vi "insertTubel.vi"(8 "error in (no error)":errorcluster, 9 "Data Cluster":T1, 10 "Name of Table":string, 11 "DataCollector in":refnum<class "DataCollector.lvclass">) -> (0 "error out":errorcluster, 3 "DataCollector out":refnum<class "DataCollector.lvclass">)   [LabVIEW 2017, in "DataCollector.lvclass"]
uses:
  DataCollector.lvclass
  DataCollector.lvclass/DataCollector.ctl
  <vilib>/drjdpowell/SQLite Library/SQL Statement/SQL Statement.lvclass/SQL Statement.ctl
  <vilib>/drjdpowell/SQLite Library/SQL Statement/Bind Integer.vi
  <vilib>/drjdpowell/SQLite Library/SQL Statement/Bind Null.vi
  <vilib>/drjdpowell/SQLite Library/SQL Statement/Step.vi
  <vilib>/drjdpowell/SQLite Library/SQL Statement/Error Message.vi
  <vilib>/drjdpowell/SQLite Library/SQL Connection/Connection.lvclass
  <vilib>/drjdpowell/SQLite Library/SQL Statement/SQL Statement.lvclass
  <vilib>/drjdpowell/SQLite Library/Transaction Helpers/Transaction.lvlib
panel:
  out "concatenated string":string
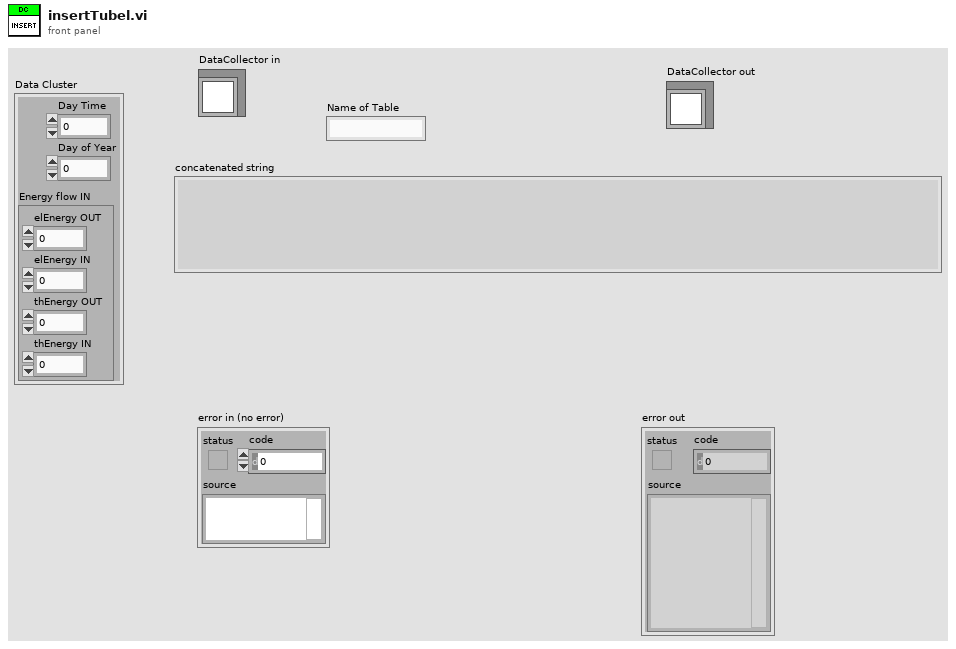
[diagram p1: front panel]
types:
  T1 = cluster{"Day Time":u32, "Day of Year":u32, "Energy flow IN":cluster{"elEnergy OUT":dbl, "elEnergy IN":dbl, "thEnergy OUT":dbl, "thEnergy IN":dbl}}
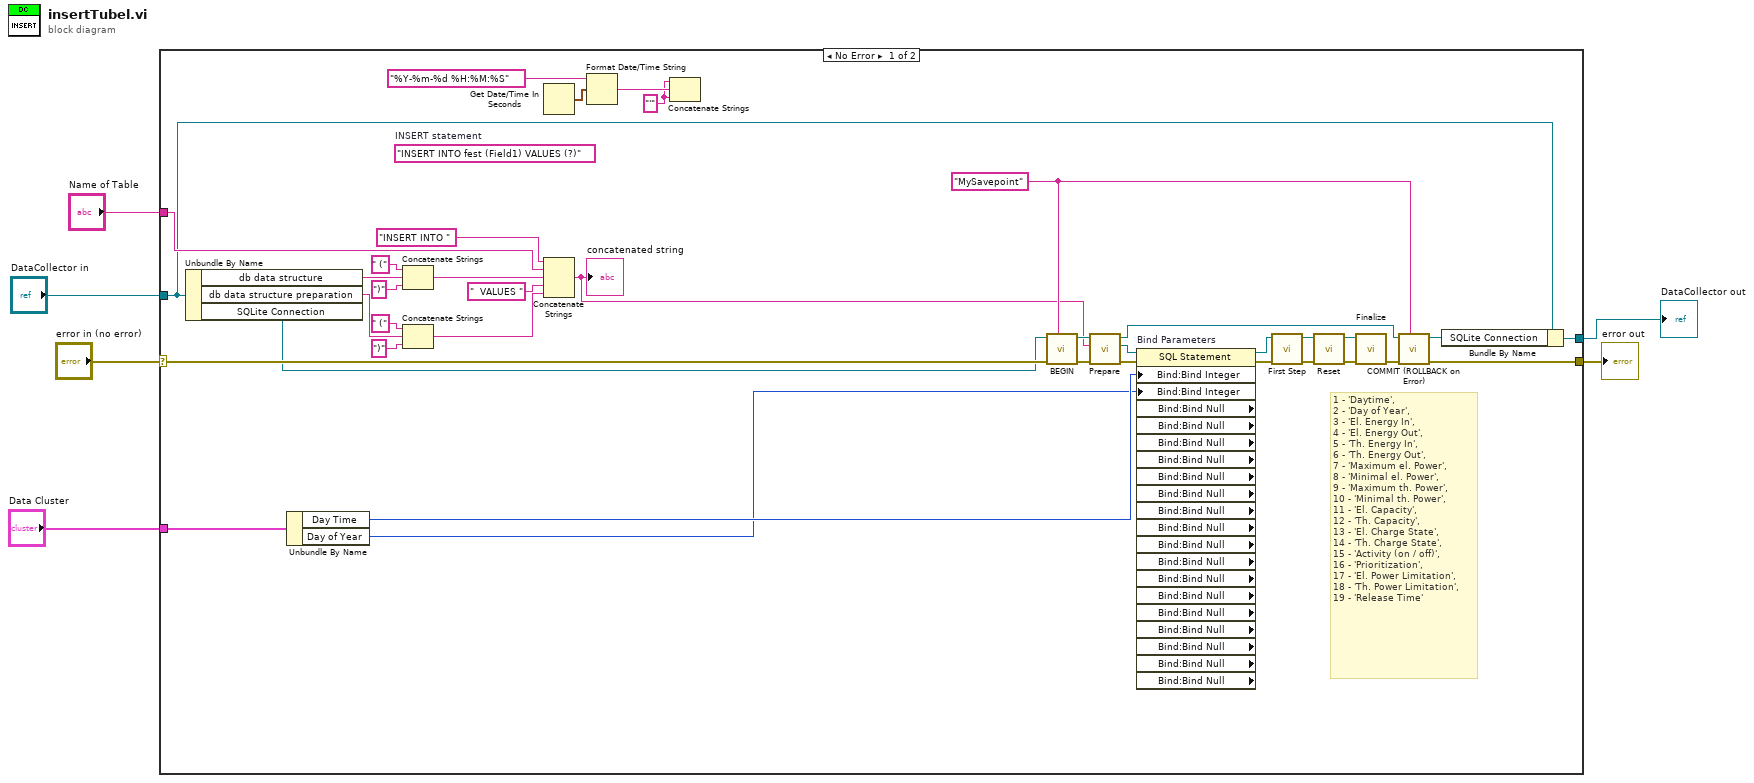
[diagram p0: block diagram]
diagram:
  n1 = case shown="No Error" "error in (no error)" {
    selector: "error in (no error)" -> [w16 w46]
    tunnel: [w15 w46] -> w4
    tunnel: [w17 w45] -> w6
    tunnel: "DataCollector in" -> [w10 w45]
    tunnel: "Name of Table" -> [w28 _]
    tunnel: "Data Cluster" -> [w9 _]
    frame No Error {
      (unwired) "INSERT INTO fest (Field1) VALUES (?)"  # INSERT statement
      w14 = "MySavepoint" ("Savepoint name")
      w43 = "'" ("String")
      # "1 - 'Daytime', \n2 - 'Day of Year', \n3 - 'El. Energy In',  \n4 - 'El. Energy Out', \n5 - 'Th. Energy In',  \n6 - 'Th. Energy Out',  \n7 - 'Maximum el. Power', \n8 - 'Minimal el. Power', \n9 - 'Maximum th. Power', \n10 - 'Minimal th. Power', \n11 - 'El. Capacity',  \n12 - 'Th. Capacity',\n13 - 'El. Charge State', \n14 - 'Th. Charge State', \n15 - 'Activity (on / off)', \n16 - 'Prioritization', \n17 - 'El. Power Limitation',  \n18 - 'Th. Power Limitation',\n19 - 'Release Time'"
      n2 = Unbundle By Name(w10) -> ("db data structure"=w24:string, "db data structure preparation"=w20:string, "SQLite Connection"=w12:refnum<class "Connection.lvclass">)
      n3 = Unbundle By Name(w9) -> ("Day Time"=w8:u32, "Day of Year"=w7:u32)
      n4 = Concatenate Strings(" (" ("string"), w24, ")" ("string")) -> (w23:string)
      n5 = Concatenate Strings(" (" ("string"), w20, ")" ("string")) -> (w19:string)
      n6 = Get Date/Time In Seconds() -> (seconds since 1Jan1904=w13:timestamp)
      n7 = Concatenate Strings("INSERT INTO " ("string"), w28, w23, "  VALUES " ("string"), w19) -> (w11:string)
      "concatenated string" <- w11
      n8 = Format Date/Time String(time format string (%c)="%Y-%m-%d %H:%M:%S" ("Zeitformatierungs-String (%c)"), seconds (now)=w13) -> (date/time string=w44:string)  [unwired: 1 in]
      n9 = Concatenate Strings(w43, w44, w43) -> ()  [unwired: 1 out]
      n10 = call <vilib>:"BEGIN.vi"("Savepoint name"=w14, "error in (no error)"=w16, "Connection in"=w12) -> ("error out"=w39:errorcluster, "Connection out"=w38:refnum<class "Connection.lvclass">)  [unwired: 7 in]
      n11 = call <vilib>:"Prepare.vi"("error in (no error)"=w39, "SQL"=w11, "SQLite Connection in"=w38) -> ("error out"=w35:errorcluster, "SQL Statement out"=w34:refnum<class "SQL Statement.lvclass">, "SQLite Connection out"=w40:refnum<class "Connection.lvclass">)  [unwired: 4 in, 2 out]
      n12 = property on="Bind Parameters" class="SQL Statement" props=["Bind:Bind Integer", "Bind:Bind Integer", "Bind:Bind Null", "Bind:Bind Null", "Bind:Bind Null", "Bind:Bind Null", "Bind:Bind Null", "Bind:Bind Null", "Bind:Bind Null", "Bind:Bind Null", "Bind:Bind Null", "Bind:Bind Null", "Bind:Bind Null", "Bind:Bind Null", "Bind:Bind Null", "Bind:Bind Null", "Bind:Bind Null", "Bind:Bind Null", "Bind:Bind Null"](reference=w34, error in=w35, "Bind:Bind Integer"=w8, "Bind:Bind Integer"=w7) -> (reference out=w33:refnum<class "SQL Statement.lvclass">, error out=w32:errorcluster)  [unwired: 17 out]
      n13 = call <vilib>:"First Step.vi"("error in (no error)"=w32, "SQL Statement in"=w33) -> ("error out"=w31:errorcluster, "SQL Statement out"=w30:refnum<class "SQL Statement.lvclass">)  [unwired: 7 in, 1 out]
      n14 = call <vilib>:"Reset.vi"("error in (no error)"=w31, "SQL Statement in"=w30) -> ("error out"=w37:errorcluster, "SQL Statement out"=w36:refnum<class "SQL Statement.lvclass">)  [unwired: 8 in]
      n15 = call <vilib>:"Finalize.vi"("error in (no error)"=w37, "SQL Statement in"=w36) -> ("error out"=w41:errorcluster)  [unwired: 9 in]
      n16 = call <vilib>:"COMMIT (ROLLBACK on Error).vi"("Savepoint name"=w14, "error in (no error)"=w41, "Connection in"=w40) -> ("error out"=w15:errorcluster, "Connection out"=w18:refnum<class "Connection.lvclass">)  [unwired: 7 in]
      n17 = Bundle By Name(cluster=w10, "SQLite Connection"=w18) -> (w17:refnum<class "DataCollector.lvclass">)
    }
    frame Error {
    }
  }
  "error out" <- w4
  "DataCollector out" <- w6
